vi "4155C PulsedStressV.vi"(0 "VISA resource name in":refnum<visa-resource-name>="GPIB0::14::INSTR", 1 "sweep mode":u16(ring) items=["Single", "Double"], 2 "Panel Controls":T4={"Emergency Stop"=refnum, "TransGraph Max"=0.001, "Text/Graph (text=false)"=FALSE, "TransGraph Min"=1e-11} {"TransGraph Min" format="%.2e"; "TransGraph Max" format="%.2e"}, 5 "Gate":T1={"Gate Start"=10.0, "Gate Stop"=0.5, "Gate Step (linear only)"=1.0, "Gate Compliance"=0.001, "Gate PComp"=0.0, "Range mode"=0, "Range"=6} {"Range" max=11 scale=0.0..11.0; "Range mode" items=["Auto", "Limited", "Fixed"]; "Gate PComp" min=0.0 max=2.0 format="%^.2e"; "Gate Compliance" min=0.0 max=0.1 format="%^.2e"; "Gate Step (linear only)" min=-100.0 max=100.0 format="%^.4e"; "Gate Stop" min=-100.0 max=100.0 format="%^.4e"; "Gate Start" min=-100.0 max=100.0 format="%^.4e"}, 7 "Drain":T6={"Drain Start"=5.0, "Drain Stop"=2.0, "Drain Compliance"=0.001, "Drain Step"=1.0, "Drain PComp"=0.0, "Range mode"=0, "Range"=6} {"Range" max=11 scale=0.0..11.0; "Range mode" items=["Auto", "Limited", "Fixed"]; "Drain PComp" min=0.0 max=2.0 format="%^.2e"; "Drain Step" min=-100.0 max=100.0 format="%^.4e"; "Drain Compliance" min=0.0 max=0.1 format="%^.2e"; "Drain Stop" min=-100.0 max=100.0 format="%^.4e"; "Drain Start" min=-100.0 max=100.0 format="%^.4e"}, 9 "Timings":T5={"integration time"=0, "Short/Long integration time"=0.00064, "hold time (sec)"=0.0, "delay time (sec)"=0.0, "Step Time (0 disables)"=0.0, "sweep method"=0, "Pulse period"=0.1, "Base voltage"=0.0, "Pulse width"=0.05} {"Pulse width" min=0.0005 max=0.1 step=0.0001 format="%.4f"; "Base voltage" min=-100.0 max=100.0 format="%^.4e"; "Pulse period" min=0.005 max=1.0 step=0.0001 format="%.4f"; "sweep method" items=["Continuous", "Pulsed"]; "Step Time (0 disables)" min=0.0 format="%.2f"; "delay time (sec)" min=0.0 format="%.4f"; "hold time (sec)" min=0.0 format="%.4f"; "Short/Long integration time" min=0.0 format="%^.0e"; "integration time" scale=0.0..2.0}, 11 "error in (no error)":errorcluster, 12 "SMU4":cluster{"on/off":bool, "Voltage":dbl} {"Voltage" min=-100.0 max=100.0 format="%.2f"}, 13 "Standby":T2) -> (4 "VISA Resource Name out":refnum<visa-resource-name>, 8 "ID":dbl[](array[numeric]) format="%.2e", 10 "IG":dbl[](array[numeric]) format="%.2e", 14 "Outparams":T3={"V2 Start"=0.0, "V2 Step"=0.0, "Number of points"=1} {"V2 Step" format="%.3f"; "V2 Start" format="%^.4e"}, 15 "error out":errorcluster)   [LabVIEW 2016]
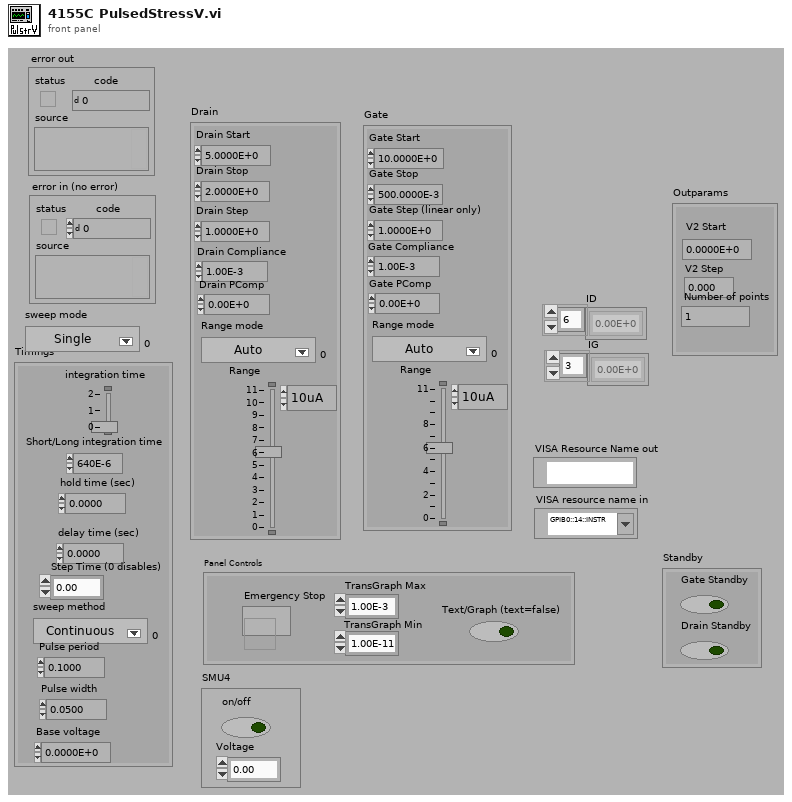
[diagram p1: front panel]
types:
  T1 = cluster{"Gate Start":dbl, "Gate Stop":dbl, "Gate Step (linear only)":dbl, "Gate Compliance":dbl, "Gate PComp":dbl, "Range mode":u16, "Range":u8}
  T2 = cluster{"Gate Standby":bool, "Drain Standby":bool}
  T3 = cluster{"V2 Start":dbl, "V2 Step":dbl, "Number of points":i32}
  T4 = cluster{"Emergency Stop":refnum<vi>, "TransGraph Max":dbl, "Text/Graph (text=false)":bool, "TransGraph Min":dbl}
  T5 = cluster{"integration time":u32, "Short/Long integration time":dbl, "hold time (sec)":dbl, "delay time (sec)":dbl, "Step Time (0 disables)":dbl, "sweep method":u16, "Pulse period":dbl, "Base voltage":dbl, "Pulse width":dbl}
  T6 = cluster{"Drain Start":dbl, "Drain Stop":dbl, "Drain Compliance":dbl, "Drain Step":dbl, "Drain PComp":dbl, "Range mode":u16, "Range":u8}
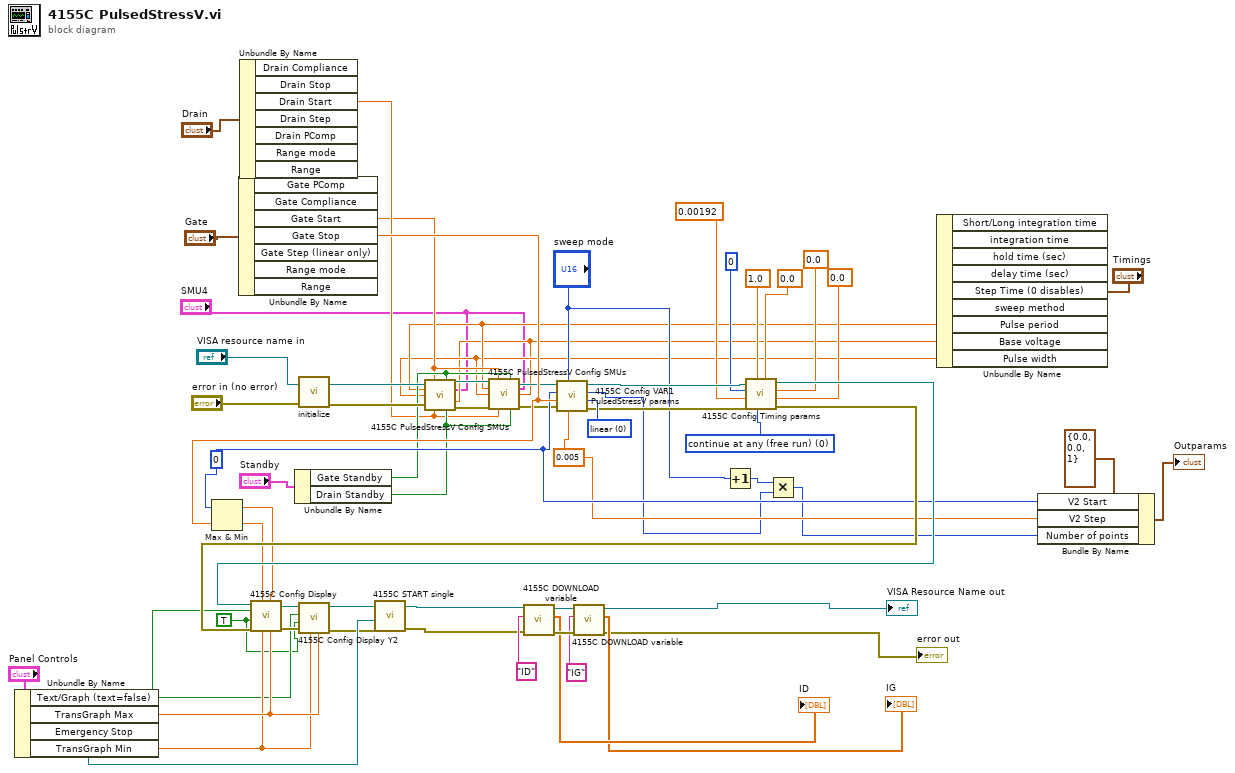
[diagram p0: block diagram]
diagram:
  w31 = 0.005 ("wait time parameter")
  w32 = 0
  w17 = TRUE ("Logarithmic")
  w58 = u8 0 items=["continue at any (free run)", "stop at any abnorm", "stop at compliance"] ("stop condition (free run:0)")
  w57 = u16 0 items=["linear", "log 10", "log 25", "log 50"] ("sweep spacing (linear: 0)")
  n1 = Unbundle By Name("Panel Controls") -> ("Text/Graph (text=false)"=w18:bool, "TransGraph Max"=w24:dbl, "Emergency Stop"=w51:refnum<vi>, "TransGraph Min"=w23:dbl)
  n2 = Unbundle By Name("Gate") -> ("Gate Start"=w5:dbl, "Gate Stop"=w38:dbl)  [unwired: 5 out]
  n3 = Max & Min(x=w32, y=w38) -> (max(x,y)=w25:dbl, min(x,y)=w26:dbl)
  n4 = Unbundle By Name("Drain") -> ("Drain Start"=w6:dbl)  [unwired: 6 out]
  n5 = Unbundle By Name("Standby") -> ("Gate Standby"=w8:bool, "Drain Standby"=w7:bool)
  n6 = call "initialize.vi"("error in (no error)"="error in (no error)", "VISA resource name in"="VISA resource name in") -> ("error out"=w14:errorcluster, "VISA Resource Name out"=w13:refnum<visa-resource-name>)
  n7 = Increment(x="sweep mode") -> (x+1=w28:u16)
  n8 = Unbundle By Name("Timings") -> ("Pulse period"=w4:dbl, "Base voltage"=w2:dbl, "Pulse width"=w3:dbl)  [unwired: 6 out]
  n9 = call "4155C PulsedStressV Config SMUs.vi"("VISA resource name in"=w13, "Gate ON voltage"=w5, "Gate Standby"=w8, "Pulse period 2"=w4, "SMU4"="SMU4", "Pulse width 2"=w3, "Base voltage 2"=w2, "error in (no error)"=w14, "Drain Voltage"=w6, "Drain Standby"=w7) -> ("VISA Resource Name out"=w9:refnum<visa-resource-name>, "error out"=w12:errorcluster)  [unwired: 4 in]
  n10 = call "4155C PulsedStressV Config SMUs.vi"("VISA resource name in"=w9, "Gate ON voltage"=w5, "Gate Standby"=w8, "Pulse period 2"=w4, "SMU4"="SMU4", "Pulse width 2"=w3, "Base voltage 2"=w2, "error in (no error)"=w12, "Drain Voltage"=w6, "Drain Standby"=w7) -> ("VISA Resource Name out"=w10:refnum<visa-resource-name>, "error out"=w11:errorcluster)  [unwired: 4 in]
  n11 = call "4155C Config VAR1 PulsedStressV params.vi"("sweep spacing (linear: 0)"=w57, "step (linear only)"=w31, "sweep mode"="sweep mode", "error in (no error)"=w11, "stop"=w38, "start"=w32, "VISA session"=w10) -> ("error out"=w39:errorcluster, "Number of points"=w29:i32, "dup VISA resource name"=w40:refnum<visa-resource-name>)  [unwired: 2 in]
  n12 = call "4155C Config Timing params.vi"("delay time (sec)"=0.0 ("wait time parameter"), "hold time (sec)"=0.0 ("wait time parameter"), "Step Time (0 disables)"=0.0 ("wait time parameter"), "stop condition (free run:0)"=w58, "wait time parameter"=1.0, "error in (no error)"=w39, "Short/Long integration time"=0.00192 ("wait time parameter"), "integration time"=0, "VISA session"=w40) -> ("error out"=w53:errorcluster, "dup VISA resource name"=w52:refnum<visa-resource-name>)  [unwired: 1 in]
  n13 = call "4155C Config Display.vi"("Ymax"=w24, "Var1 Stop"=w25, "Ymin"=w23, "Var1 Start"=w26, "error in (no error)"=w53, "Logarithmic"=w17, "SPA Display"=w18, "VISA session"=w52) -> ("error out"=w22:errorcluster, "dup VISA resource name"=w19:refnum<visa-resource-name>)  [unwired: 2 in]
  n14 = call "4155C Config Display Y2.vi"("Ymax"=w24, "Ymin"=w23, "error in (no error)"=w22, "Logarithmic"=w17, "SPA Display"=w18, "VISA session"=w19) -> ("error out"=w21:errorcluster, "dup VISA resource name"=w20:refnum<visa-resource-name>)  [unwired: 4 in]
  n15 = call "4155C START single.vi"("error in (no error)"=w21, "Emergency Stop"=w51, "VISA resource name in"=w20) -> ("error out"=w45:errorcluster, "VISA Resource Name out"=w46:refnum<visa-resource-name>)  [unwired: 3 in]
  n16 = call "4155C DOWNLOAD variable.vi"("error in (no error)"=w45, "Variable name"="ID", "VISA resource name in"=w46) -> ("error out"=w63:errorcluster, "Output data"=→"ID":dbl[], "VISA Resource Name out"=w62:refnum<visa-resource-name>)  [unwired: 2 in]
  n17 = call "4155C DOWNLOAD variable.vi"("error in (no error)"=w63, "Variable name"="IG", "VISA resource name in"=w62) -> ("error out"=→"error out":errorcluster, "Output data"=→"IG":dbl[], "VISA Resource Name out"=→"VISA Resource Name out":refnum<visa-resource-name>)  [unwired: 2 in]
  n18 = Multiply(x=w28, y=w29) -> (x*y=w27:i32)
  n19 = Bundle By Name(cluster=T3 {"V2 Start"=0.0, "V2 Step"=0.0, "Number of points"=1} ("Outparams"), "V2 Start"=w32, "V2 Step"=w31, "Number of points"=w27) -> (→"Outparams":T3)
